vi "User Example.vi"() -> ()   [LabVIEW 2019, in "xy_utilities.lvlib"]
uses:
  User.Example/User.Example.lvclass
  C:/Users/patrick/Documents/GitHub/ciozi137/XY-Utilities/src/User/User.lvclass
  User/User.lvclass
  User/User (single).vi
  xy_utilities.lvlib
panel:
  out "error out":errorcluster
  out "XY-data out":cluster{"X-array":dbl[], "Y-array":dbl[]} {"Y-array" format="%.2p"; "X-array" format="%.2p"}
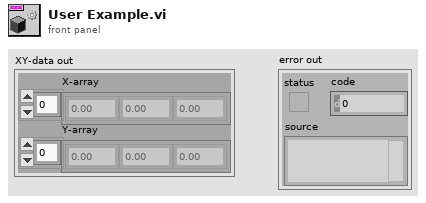
[diagram p1: front panel]
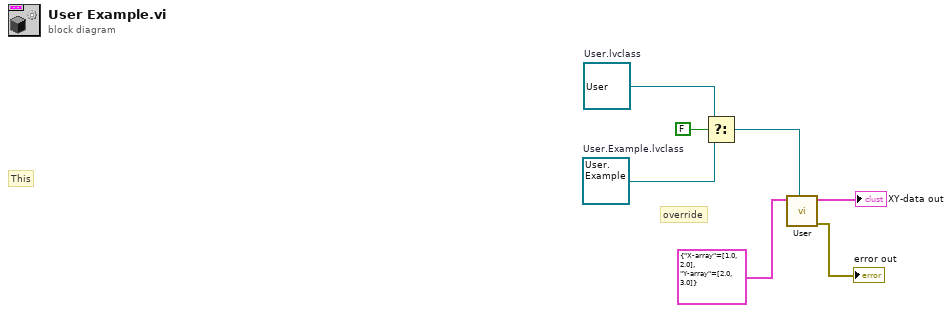
[diagram p0: block diagram]
diagram:
  w4 = refnum<class "User.lvclass"> refnum  # User.lvclass
  w3 = refnum<class "User.Example.lvclass"> refnum  # User.Example.lvclass
  # "override"
  # "This"
  n1 = Select(t=w4, s=FALSE, f=w3) -> (s? t:f=w1:refnum<class "User.lvclass">)
  n2 = call-poly "User.vi"("User.lvclass"=w1, "XY-data"=cluster{"X-array":dbl[], "Y-array":dbl[]} {"X-array"=[1.0, 2.0], "Y-array"=[2.0, 3.0]}) -> ("error out"=→"error out":errorcluster, "XY-data out"=→"XY-data out":cluster{"X-array":dbl[], "Y-array":dbl[]})  [unwired: 7 in, 1 out]
